vi "InsertPanelToMainframe.vi"(8 "error in (no error)":errorcluster, 9 "VI Refnum":refnum<vi>, 10 "Sub Panel":string, 11 "Microscope Controller in":refnum<class "MicroscopeController.lvclass">) -> (0 "error out":errorcluster, 3 "Microscope Controller out":refnum<class "MicroscopeController.lvclass">)   [LabVIEW 2020, in "MicroscopeController.lvlib" / "MicroscopeController.lvclass"]
uses:
  MicroscopeController.lvclass
  MicroscopeController.lvclass/MicroscopeController.ctl
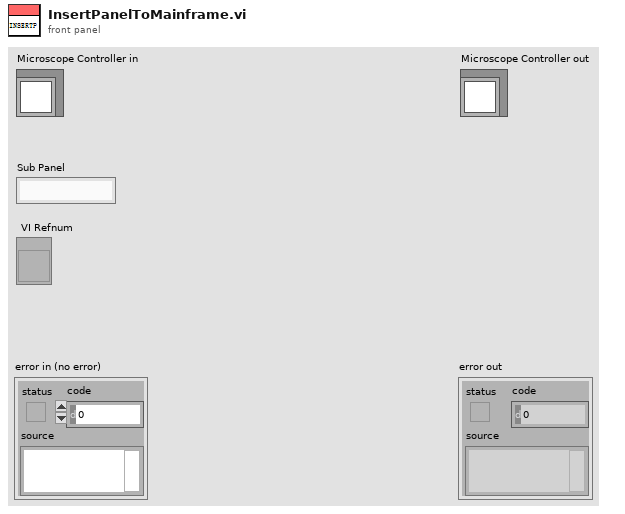
[diagram p1: front panel]
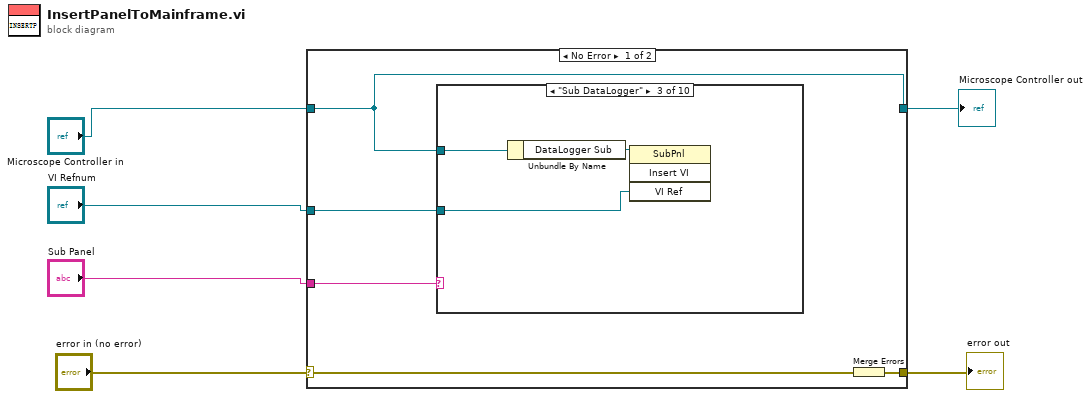
[diagram p0: block diagram]
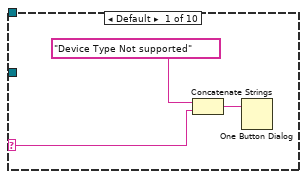
[diagram p2: hidden frame]
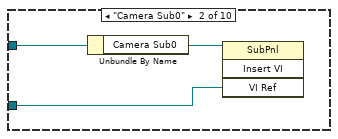
[diagram p3: hidden frame]
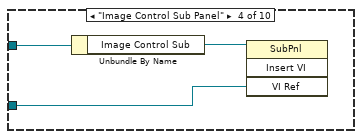
[diagram p4: hidden frame]
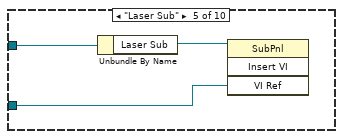
[diagram p5: hidden frame]
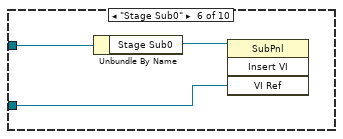
[diagram p6: hidden frame]
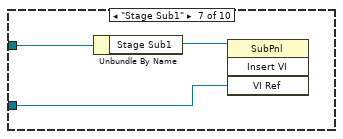
[diagram p7: hidden frame]
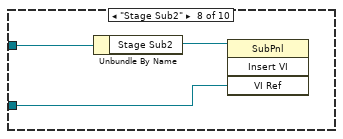
[diagram p8: hidden frame]
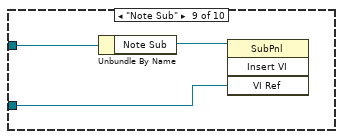
[diagram p9: hidden frame]
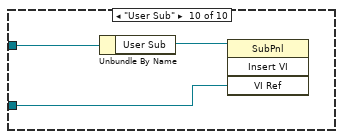
[diagram p10: hidden frame]
diagram:
  n1 = case shown="No Error" "error in (no error)" {
    selector: "error in (no error)" -> [w10 w43]
    tunnel: [w9 w43] -> w1
    tunnel: [w11 w42] -> w3
    tunnel: "Microscope Controller in" -> [w11 w42]
    tunnel: "VI Refnum" -> [w8 _]
    tunnel: "Sub Panel" -> [w7 _]
    frame No Error {
      n2 = case shown="\"Sub DataLogger\"" w7 {
        selector: w7 -> [w13 _ _ _ _ _ _ _ _ _]
        tunnel: w11 -> [_ w17 w20 w23 w26 w29 w32 w35 w38 w41]
        tunnel: w8 -> [_ w15 w18 w21 w24 w27 w30 w33 w36 w39]
        frame Default {
          n3 = Concatenate Strings("Device Type Not supported" ("string"), w13) -> (w14:string)
          n4 = One Button Dialog(message=w14) -> ()  [unwired: 1 in, 1 out]
        }
        frame "Camera Sub0" {
          n5 = Unbundle By Name(w17) -> ("Camera Sub0"=w16:refnum<vi>)
          n6 = invoke class="SubPnl" method="Insert VI"(reference=w16, "VI Ref"=w15) -> ()  [unwired: 2 in, 4 out]
        }
        frame "Sub DataLogger" {
          n7 = Unbundle By Name(w20) -> ("DataLogger Sub"=w19:refnum<vi>)
          n8 = invoke class="SubPnl" method="Insert VI"(reference=w19, "VI Ref"=w18) -> ()  [unwired: 2 in, 4 out]
        }
        frame "Image Control Sub Panel" {
          n9 = Unbundle By Name(w23) -> ("Image Control Sub"=w22:refnum<vi>)
          n10 = invoke class="SubPnl" method="Insert VI"(reference=w22, "VI Ref"=w21) -> ()  [unwired: 2 in, 4 out]
        }
        frame "Laser Sub" {
          n11 = Unbundle By Name(w26) -> ("Laser Sub"=w25:refnum<vi>)
          n12 = invoke class="SubPnl" method="Insert VI"(reference=w25, "VI Ref"=w24) -> ()  [unwired: 2 in, 4 out]
        }
        frame "Stage Sub0" {
          n13 = Unbundle By Name(w29) -> ("Stage Sub0"=w28:refnum<vi>)
          n14 = invoke class="SubPnl" method="Insert VI"(reference=w28, "VI Ref"=w27) -> ()  [unwired: 2 in, 4 out]
        }
        frame "Stage Sub1" {
          n15 = Unbundle By Name(w32) -> ("Stage Sub1"=w31:refnum<vi>)
          n16 = invoke class="SubPnl" method="Insert VI"(reference=w31, "VI Ref"=w30) -> ()  [unwired: 2 in, 4 out]
        }
        frame "Stage Sub2" {
          n17 = Unbundle By Name(w35) -> ("Stage Sub2"=w34:refnum<vi>)
          n18 = invoke class="SubPnl" method="Insert VI"(reference=w34, "VI Ref"=w33) -> ()  [unwired: 2 in, 4 out]
        }
        frame "Note Sub" {
          n19 = Unbundle By Name(w38) -> ("Note Sub"=w37:refnum<vi>)
          n20 = invoke class="SubPnl" method="Insert VI"(reference=w37, "VI Ref"=w36) -> ()  [unwired: 2 in, 4 out]
        }
        frame "User Sub" {
          n21 = Unbundle By Name(w41) -> ("User Sub"=w40:refnum<vi>)
          n22 = invoke class="SubPnl" method="Insert VI"(reference=w40, "VI Ref"=w39) -> ()  [unwired: 2 in, 4 out]
        }
      }
      n23 = Merge Errors(w10) -> (w9:errorcluster)
    }
    frame Error {
    }
  }
  "error out" <- w1
  "Microscope Controller out" <- w3
